vi "RT Main and Scoreboard.vi"() -> ()   [LabVIEW 2026]
uses:
  RT Image.ctl
  RT States.ctl
  Idle Pattern.ctl
  Score.ctl
  SideSelector.ctl
  RT Commands.ctl
  Game Settings.ctl
  2 Player Bitfile dynRef.ctl
  <vilib>/FPGAPlugInAG/cRIO-9047/niLvFpga_Open_cRIO-9047.vi
  <vilib>/rvi/interface/common/dynamic/niFpgaDynamicAddResources.vi
  <vilib>/FPGAPlugInAG/Dynamic/niLvFpga_Run_Dynamic.vi
  <vilib>/Utility/error.llb/Error Cluster From Error Code.vi
  <vilib>/rvi/errors/niLvFpgaAdjustHostInterfaceError.vi
  <vilib>/FPGAPlugInAG/Dynamic/niLvFpga_Abort_Dynamic.vi
  <vilib>/FPGAPlugInAG/Dynamic/niLvFpga_Close_Dynamic.vi
  <vilib>/rvi/interface/nirviOpenFPGA/nirviOpenFPGA.xnode
  FPGA Bitfiles/speedofvight_IdlePattern.lvbitx
  <vilib>/rvi/interface/nirviMethod/nirviMethod.xnode
  <vilib>/rvi/interface/nirviReadWriteControl/nirviReadWriteControl.xnode
  <vilib>/rvi/interface/nirviCloseFPGA/nirviCloseFPGA.xnode
  FPGA Bitfiles/speedofvight_1Player.lvbitx
  FPGA Bitfiles/speedofvight_2Player.lvbitx
  <vilib>/rvi/interface/Simulation/niFpgaSimulationCallBeginRW.vi
  NiFpgaLv.dll
  <vilib>/Utility/Data Type/NI_Data Type.lvlib
panel:
  out "error out 3":errorcluster
  out "error out 2":errorcluster
  out "x-y*floor(x/y)":u32
  out "floor(x/y)":u32
  in  "Winner Display time, ms":u32=7000
  in  "2 Players":bool
  in  "Idle Pattern Cycle Time":u32=5000
  in  "abort":bool
  in  "End Idle":bool
  out "error out":errorcluster
  in  "Speed Threshold, ticks":u64=3000
  in  "Debounce Threshold, ticks":u64=5000
  in  "Game Time":u32=4
  in  "End Game":bool
  out "Score P1":u16 format="%03.0f"
  out "Score P2":u16 format="%03.0f"
  out "2D Picture":T1
  out "Time Remaining":u32 format="%03.0f"
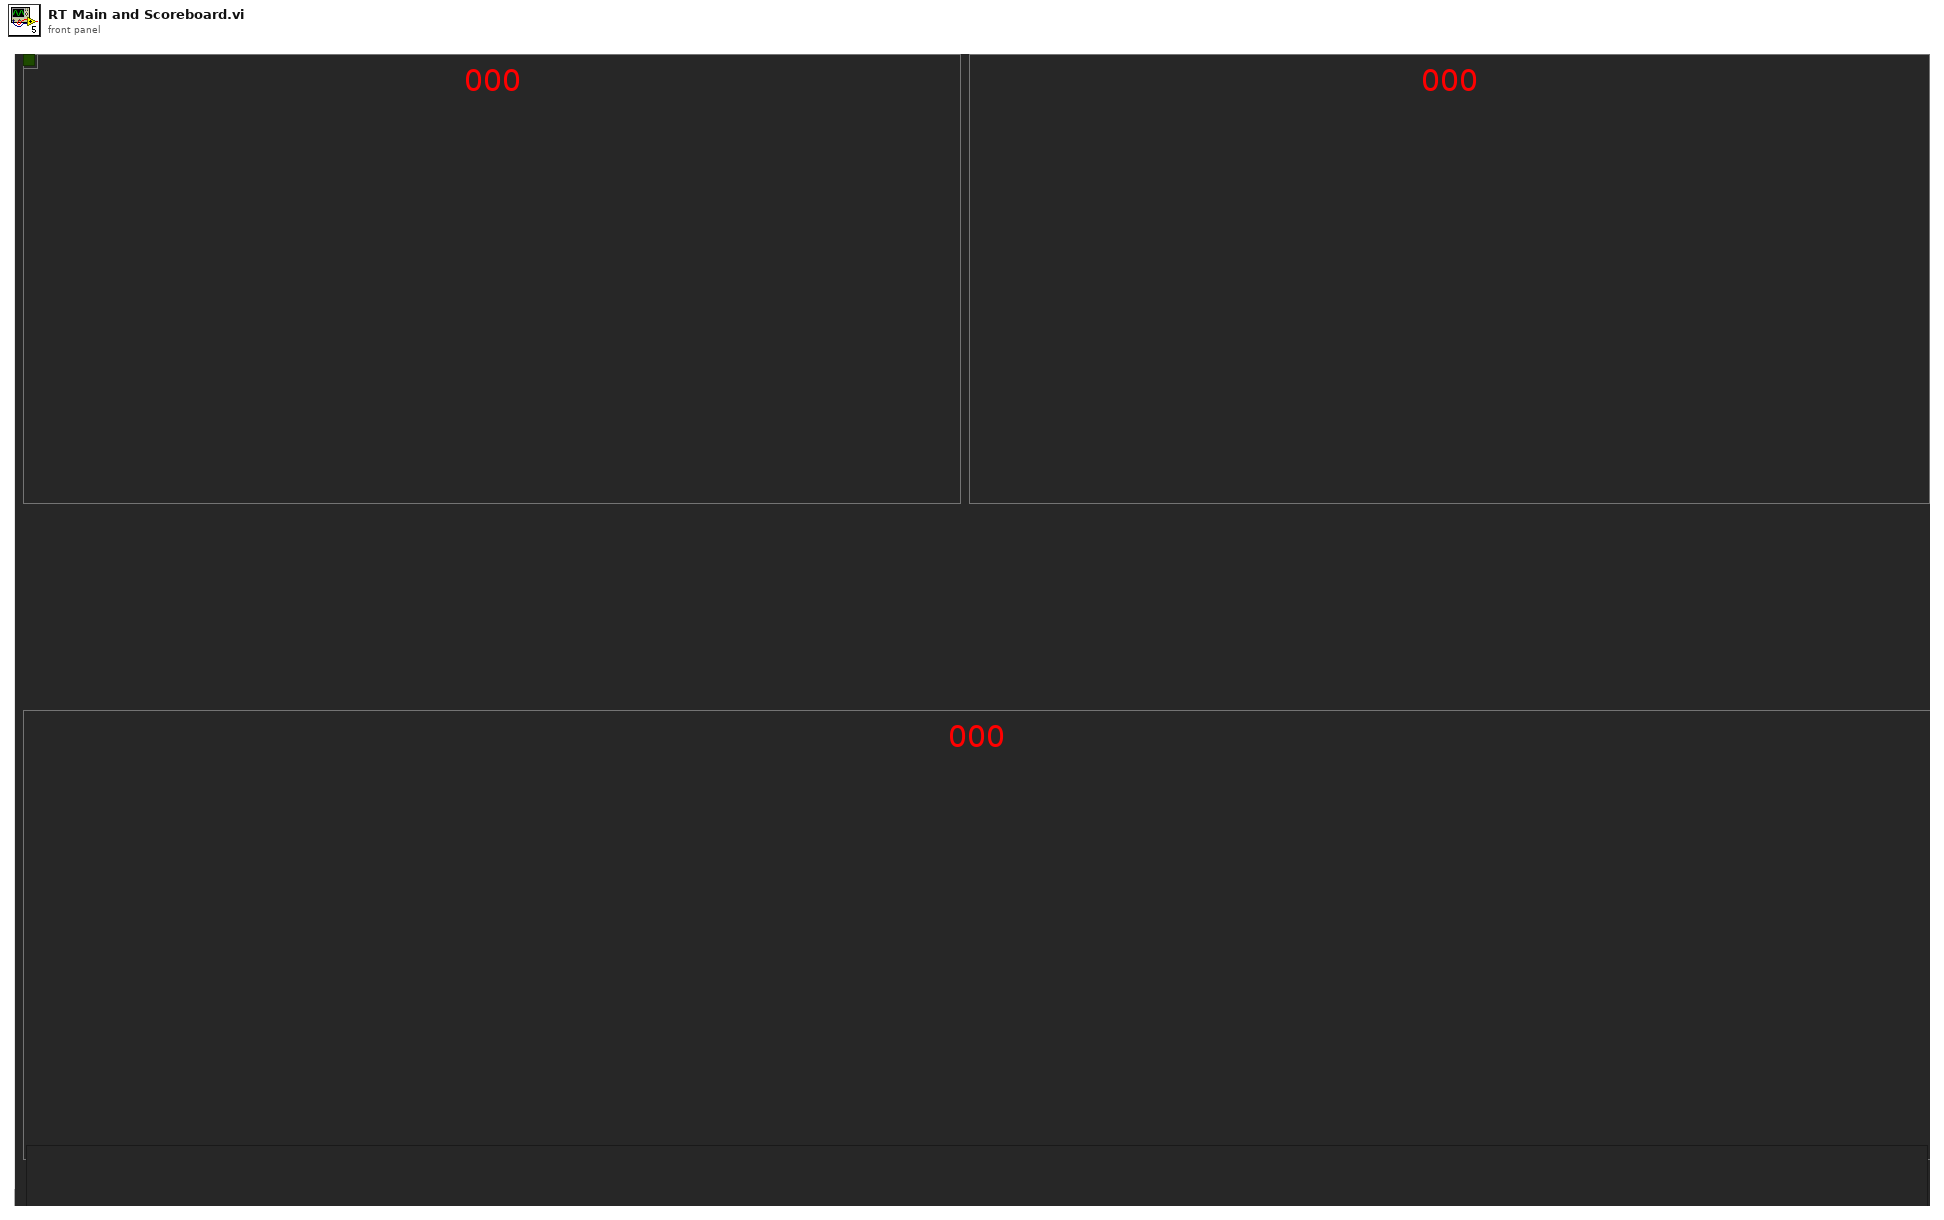
[diagram p1: front panel]
types:
  T1 = typedef "RT Image.ctl" = picture
  T2 = typedef "Score.ctl" = cluster{"Score P1":u16, "Score P2":u16, "Winner Selection":T3}
  T3 = typedef "SideSelector.ctl" = enum16{"P12", "P1", "P2"}
  T4 = cluster{"Debounce Threshold, ticks":u64, "Speed Threshold, ticks":u64, "Game Time":u32, "Idle Pattern Cycle Time, ms":u32, "Winner Display time, ms":u32, "Final Score":T2}
  T5 = typedef "Idle Pattern.ctl" = enum16{"Expanding Circle", "Plasma", "Radar Sweep", "Matrix Rain", "Campfire", "Diagonal Scan"}
  T6 = typedef "RT States.ctl" = enum16{"Idle", "Configuring", "1Player", "2Player", "Display Winner"}
  T7 = typedef "RT Commands.ctl" = enum16{"<null>", "End Idle", "Reset", "Commit Settings", "Commit Host Settings"}
  T8 = typedef "2 Player Bitfile dynRef.ctl" = refnum<k20>
  T9 = typedef "Game Settings.ctl" = cluster{"Speed Threshold, ticks":u64, "Game Time":u32, "2 Players":bool}
  T10 = cluster{"Score P1":u16, "Score P2":u16, "Winner Selection":T3}
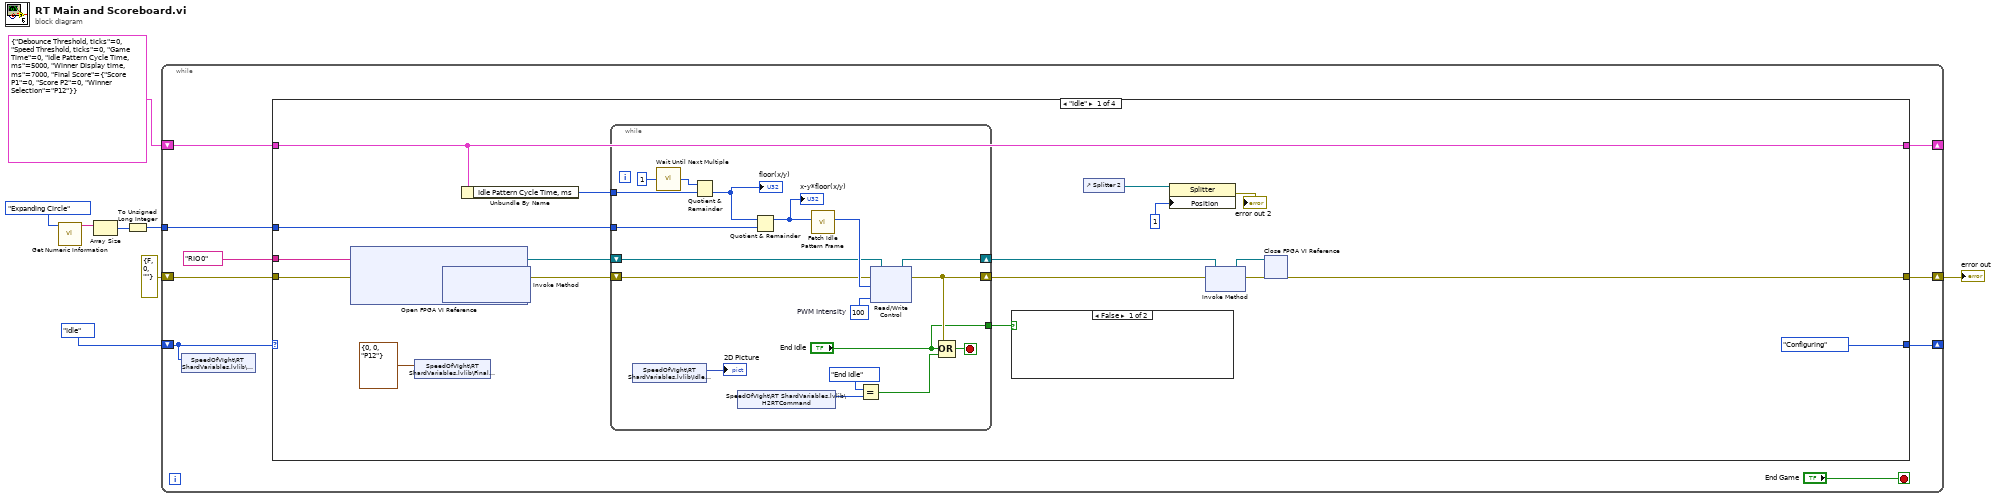
[diagram p0: block diagram]
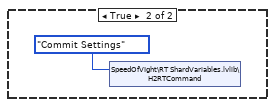
[diagram p2: hidden frame]
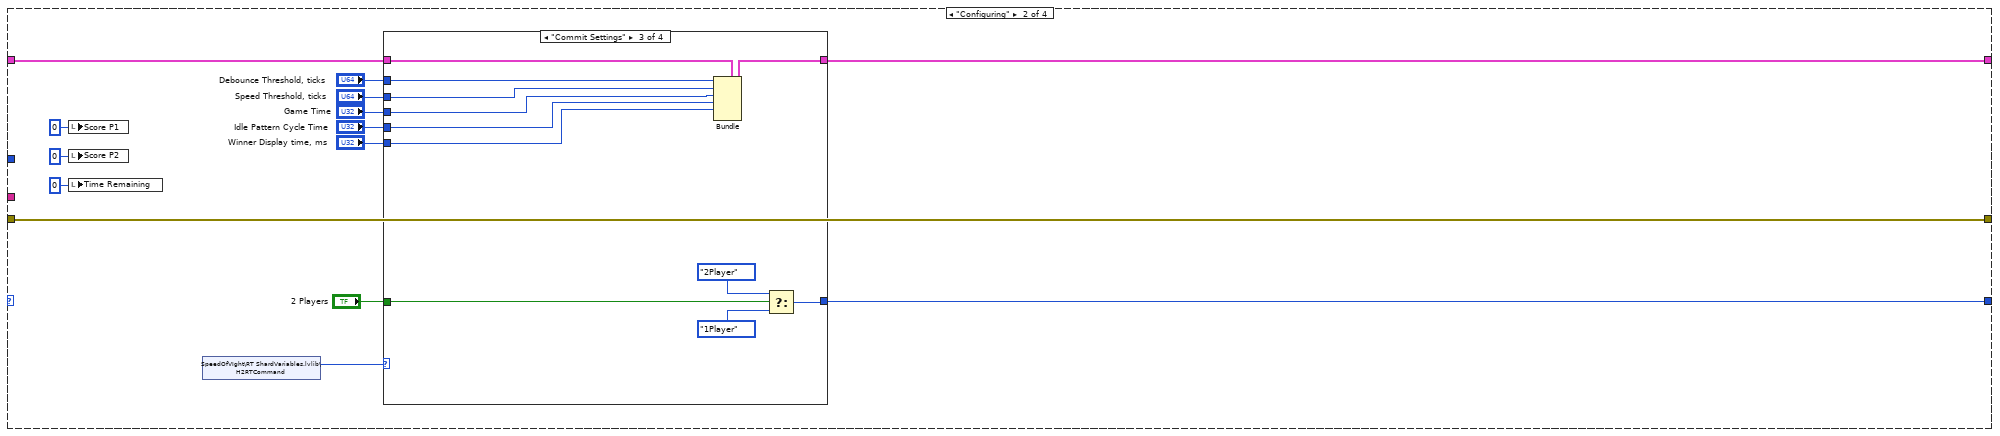
[diagram p3: hidden frame]
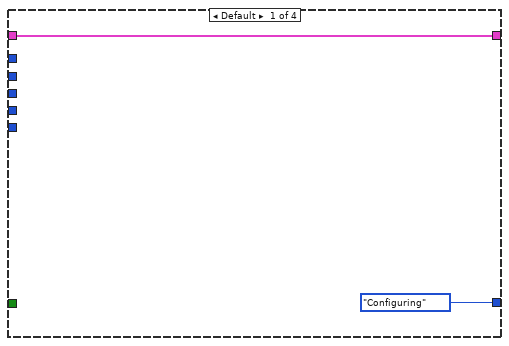
[diagram p4: hidden frame]
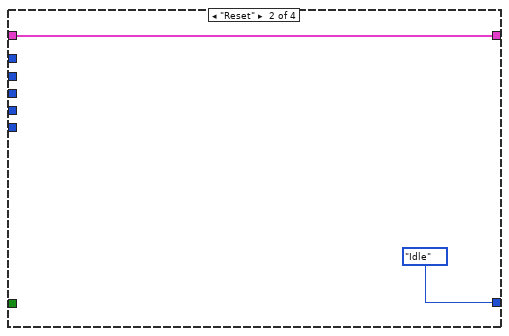
[diagram p5: hidden frame]
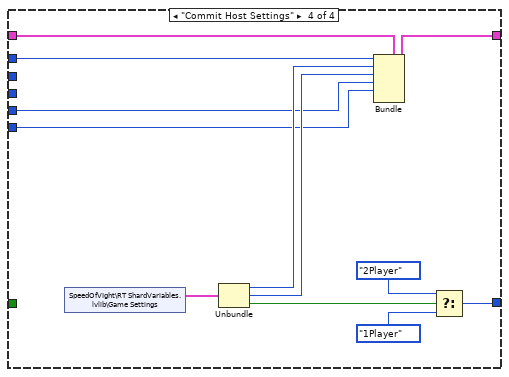
[diagram p6: hidden frame]
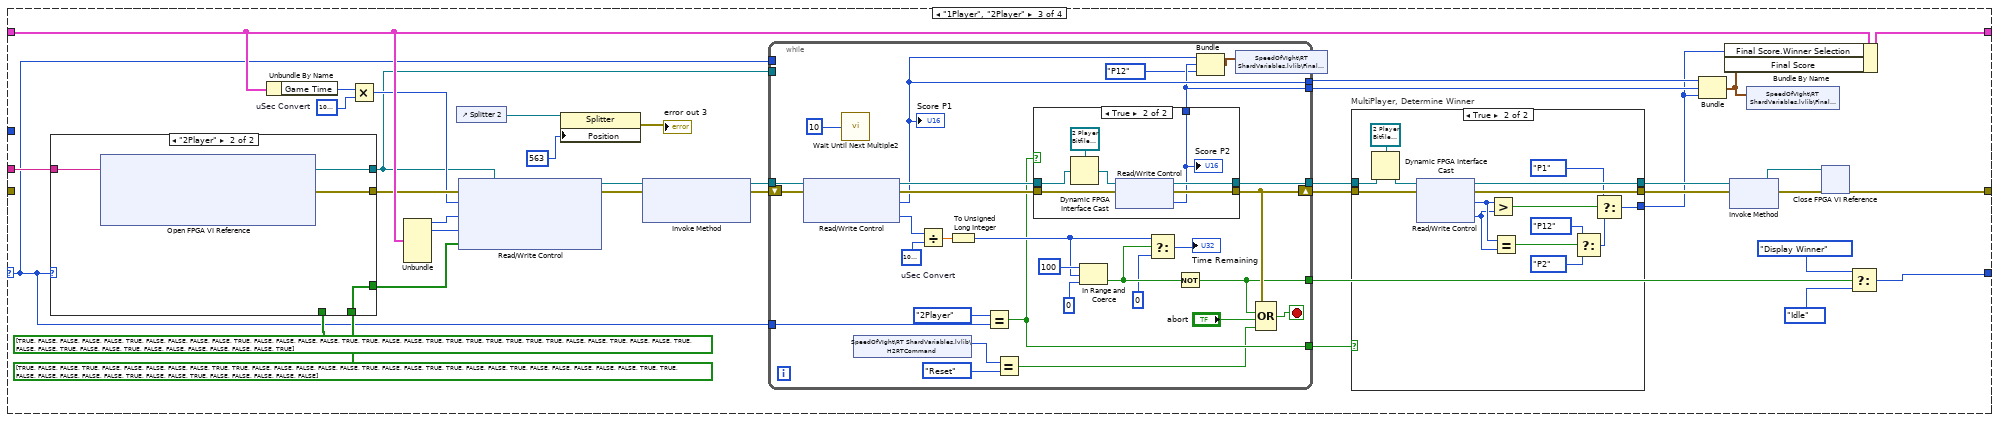
[diagram p7: hidden frame]
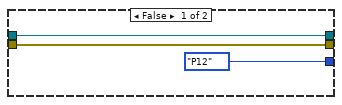
[diagram p8: hidden frame]
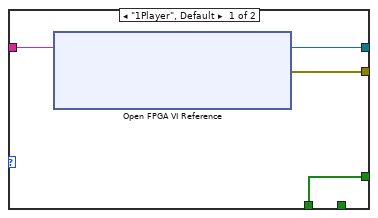
[diagram p9: hidden frame]
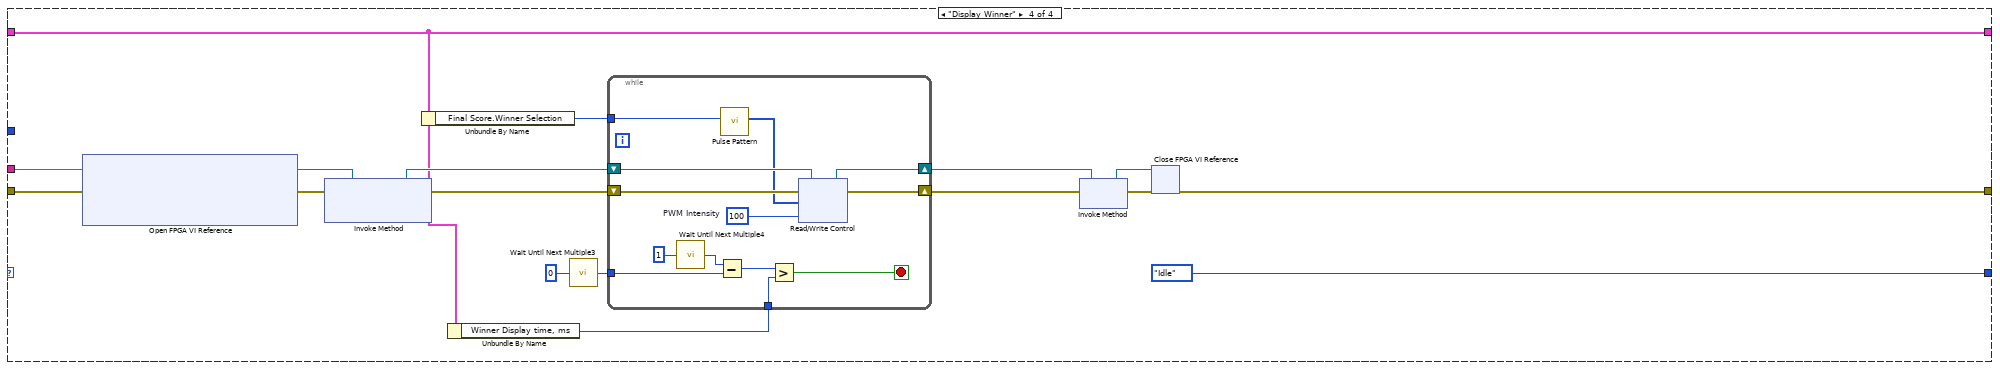
[diagram p11: hidden frame]
diagram:
  n1 = call <vilib>:"Get Numeric Information.vi"("variant"=Idle_Pattern."Expanding Circle" ("Effect")) -> ("enum names"=w6:string[])  [unwired: 7 in, 3 out]
  n2 = Array Size(array=w6) -> (size(s)=w5:i32)
  n3 = To Unsigned Long Integer(number=w5) -> (unsigned 32bit integer=w1:u32)
  n4 = while {
    shift-right: [w13] -> _
    shift-left: RT_States."Idle" ("Enum") -> [w10]
    tunnel: w1 -> [w16]
    shift-right: [w15] -> w4
    shift-left: errorcluster {"status"=FALSE, "code"=0, "source"=""} ("error out") -> [w14]
    shift-right: [w11] -> _
    shift-left: T4 {"Debounce Threshold, ticks"=0, "Speed Threshold, ticks"=0, "Game Time"=0, "Idle Pattern Cycle Time, ms"=5000, "Winner Display time, ms"=7000, "Final Score"={"Score P1"=0, "Score P2"=0, "Winner Selection"=enum."P12"}} ("cluster") -> [w12]
    stop <- "End Game" stop-if-true
    n5 = shared-variable "SpeedOfVIght\\RT ShardVariables.lvlib\\RT2HState"(w10) -> ()  [unwired: 1 in, 1 out]
    n6 = case shown="\"Idle\"" w10 {
      selector: w10 -> [_ _ w103 _]
      tunnel: tag "RIO0" ("resource name") -> [w33 _ w126 w211]
      tunnel: w16 -> [w32 _ _ _]
      tunnel: [w27 w70 w120 w206] -> w15
      tunnel: w14 -> [w26 w70 _ w205]
      tunnel: [RT_States."Configuring" ("Enum") w67 w113 RT_States."Idle" ("Enum")] -> w13
      tunnel: w12 -> [w23 w69 w134 w199]
      tunnel: [w23 w68 w114 w199] -> w11
      frame "Idle" {
        n7 = xnode "Open FPGA VI Reference"("error in"=w26, "resource name"=w33) -> ("FPGA VI Reference Out"=w35:refnum<k20>, "error out"=w37:errorcluster)
        n8 = shared-variable "SpeedOfVIght\\RT ShardVariables.lvlib\\Final Score"(T2 {"Score P1"=0, "Score P2"=0, "Winner Selection"=enum."P12"} ("Final Score")) -> ()  [unwired: 1 in, 1 out]
        n9 = xnode "Invoke Method"("FPGA VI Reference In"=w35, "error in"=w37) -> ("FPGA VI Reference Out"=w34:refnum<k20>, "error out"=w36:errorcluster)  [unwired: 1 in]
        n10 = Unbundle By Name(w23) -> ("Idle Pattern Cycle Time, ms"=w24:u32)
        n11 = while {
          shift-right: [w47] -> w29
          shift-left: w36 -> [w54]
          shift-right: [w52] -> w28
          shift-left: w34 -> [w53]
          tunnel: w32 -> [w45]
          tunnel: w24 -> [w46]
          tunnel: ["End Idle"] -> w22
          stop <- w50 stop-if-true
          w55 = u16 100  # PWM Intensity
          n12 = shared-variable "SpeedOfVIght\\RT ShardVariables.lvlib\\Idle Image"() -> (→"2D Picture":T1)  [unwired: 1 in, 1 out]
          n13 = call "Wait Until Next Multiple"("Count(mSec)"=u32 1 ("Count(Ticks)")) -> ("Tick Count(mSec)"=w42:u32)
          n14 = Quotient & Remainder(x=w42, y=w46) -> (floor(x/y)=w44:u32)  [unwired: 1 out]
          "floor(x/y)" <- w44
          n15 = shared-variable "SpeedOfVIght\\RT ShardVariables.lvlib\\H2RTCommand"() -> (w41:T7)  [unwired: 1 in, 1 out]
          n16 = Quotient & Remainder(x=w44, y=w45) -> (x-y*floor(x/y)=w43:u32)  [unwired: 1 out]
          "x-y*floor(x/y)" <- w43
          n17 = call "Fetch Idle Pattern Frame.vi"("Effect"=w43) -> ("Array"=w56:u16[])  [unwired: 10 in]
          n18 = Equal?(x=RT_Commands."End Idle", y=w41) -> (x = y?=w48:bool)
          n19 = xnode "Read/Write Control"("FPGA VI Reference In"=w53, "error in"=w54, "x"=w56, "Period"=w55) -> ("FPGA VI Reference Out"=w52:refnum<k20>, "error out"=w47:errorcluster)
          n20 = Compound Arithmetic op=OR(w47, "End Idle", w48) -> (w50:bool)
        }
        n21 = case shown="False" w22 {
          frame False {
          }
          frame True {
            n22 = shared-variable "SpeedOfVIght\\RT ShardVariables.lvlib\\H2RTCommand"(RT_Commands."Commit Settings" ("H2RTCommand")) -> ()  [unwired: 1 in, 1 out]
          }
        }
        n23 = control-ref of="Splitter 2"() -> (w20:refnum<vi>)
        n24 = property class="Splitter"(reference=w20, "Position"=1 ("Splitter Position")) -> (error out=→"error out 2":errorcluster)  [unwired: 1 in, 1 out]
        n25 = xnode "Invoke Method"("FPGA VI Reference In"=w28, "error in"=w29) -> ("FPGA VI Reference Out"=w31:refnum<k20>, "error out"=w30:errorcluster)
        n26 = xnode "Close FPGA VI Reference"("FPGA VI Reference In"=w31, "error in"=w30) -> ("error out"=w27:errorcluster)
      }
      frame "Configuring" {
        n27 = local write "Score P1"(u16 0 ("Score P1")) -> ()
        n28 = local write "Score P2"(u16 0 ("Score P2")) -> ()
        n29 = local write "Time Remaining"(u32 0 ("Time Remaining")) -> ()
        n30 = shared-variable "SpeedOfVIght\\RT ShardVariables.lvlib\\H2RTCommand"() -> (w63:T7)  [unwired: 1 in, 1 out]
        n31 = case shown="\"Commit Settings\"" w63 {
          tunnel: w69 -> [w71 w74 w83 w95]
          tunnel: [w71 w74 w82 w94] -> w68
          tunnel: [RT_States."Configuring" ("Enum") RT_States."Idle" ("Enum") w81 w93] -> w67
          tunnel: "Winner Display time, ms" -> [_ _ w75 w86]
          tunnel: "Idle Pattern Cycle Time" -> [_ _ w76 w87]
          tunnel: "Speed Threshold, ticks" -> [_ _ w80 _]
          tunnel: "Debounce Threshold, ticks" -> [_ _ w79 w92]
          tunnel: "Game Time" -> [_ _ w78 _]
          tunnel: "2 Players" -> [_ _ w77 _]
          frame Default {
          }
          frame "Reset" {
          }
          frame "Commit Settings" {
            n32 = Bundle(cluster=w83, "Debounce Threshold, ticks"=w79, "Speed Threshold, ticks"=w80, "Game Time"=w78, "Idle Pattern Cycle Time, ms"=w76, "Winner Display time, ms"=w75) -> (w82:T4)  [unwired: 1 in]
            n33 = Select(t=RT_States."2Player" ("Enum"), s=w77, f=RT_States."1Player" ("Enum")) -> (s? t:f=w81:T6)
          }
          frame "Commit Host Settings" {
            n34 = shared-variable "SpeedOfVIght\\RT ShardVariables.lvlib\\Game Settings"() -> (w91:T9)  [unwired: 1 in, 1 out]
            n35 = Unbundle(w91) -> ("Speed Threshold, ticks"=w90:u64, "Game Time"=w88:u32, "2 Players"=w89:bool)
            n36 = Bundle(cluster=w95, "Debounce Threshold, ticks"=w92, "Speed Threshold, ticks"=w90, "Game Time"=w88, "Idle Pattern Cycle Time, ms"=w87, "Winner Display time, ms"=w86) -> (w94:T4)  [unwired: 1 in]
            n37 = Select(t=RT_States."2Player" ("Enum"), s=w89, f=RT_States."1Player" ("Enum")) -> (s? t:f=w93:T6)
          }
        }
      }
      frame "1Player", "2Player" {
        w133 = u32 1000000  # uSec Convert
        n38 = case shown="\"2Player\"" w103 {
          tunnel: [w156 w160] -> w130
          tunnel: [w155 w159] -> w102
          tunnel: w126 -> [w154 w158]
          tunnel: [w153 w157] -> w101
          tunnel: bool[] [TRUE, FALSE, FALSE, TRUE, FALSE, FALSE, FALSE, FALSE, FALSE, TRUE, TRUE, FALSE, FALSE, FALSE, FALSE, FALSE, TRUE, FALSE, FALSE, TRUE, TRUE, FALSE, FALSE, TRUE, FALSE, FALSE, FALSE, FALSE, FALSE, TRUE, TRUE, FALSE, FALSE, FALSE, FALSE, FALSE, TRUE, FALSE, FALSE, TRUE, FALSE, FALSE, FALSE, FALSE, FALSE] ("appended array") -> [_ w157]
          tunnel: bool[] [TRUE, FALSE, FALSE, FALSE, FALSE, TRUE, FALSE, FALSE, FALSE, FALSE, TRUE, FALSE, FALSE, FALSE, FALSE, TRUE, TRUE, FALSE, FALSE, TRUE, TRUE, TRUE, TRUE, TRUE, TRUE, TRUE, FALSE, FALSE, TRUE, FALSE, FALSE, TRUE, FALSE, FALSE, TRUE, FALSE, FALSE, TRUE, FALSE, FALSE, FALSE, FALSE, FALSE, FALSE, TRUE] ("appended array") -> [w153 _]
          frame "1Player", Default {
            n39 = xnode "Open FPGA VI Reference"("resource name"=w154) -> ("FPGA VI Reference Out"=w155:refnum<k20>, "error out"=w156:errorcluster)  [unwired: 1 in]
          }
          frame "2Player" {
            n40 = xnode "Open FPGA VI Reference"("resource name"=w158) -> ("FPGA VI Reference Out"=w159:refnum<k20>, "error out"=w160:errorcluster)  [unwired: 1 in]
          }
        }
        n41 = Unbundle By Name(w134) -> ("Game Time"=w123:u32)
        n42 = Multiply(x=w123, y=w133) -> (x*y=w127:u32)
        n43 = Unbundle(w134) -> ("Debounce Threshold, ticks"=w125:u64, "Speed Threshold, ticks"=w124:u64)  [unwired: 4 out]
        n44 = control-ref of="Splitter 2"() -> (w100:refnum<vi>)
        n45 = xnode "Read/Write Control"("FPGA VI Reference In"=w102, "error in"=w130, "Game Time, uS"=w127, "Debounce Threshold, ticks"=w125, "Speed Threshold, ticks"=w124, "Starting Lights"=w101) -> ("FPGA VI Reference Out"=w128:refnum<k20>, "error out"=w129:errorcluster)
        n46 = property class="Splitter"(reference=w100, "Position"=563 ("Splitter Position")) -> (error out=→"error out 3":errorcluster)  [unwired: 1 in, 1 out]
        n47 = xnode "Invoke Method"("FPGA VI Reference In"=w128, "error in"=w129) -> ("FPGA VI Reference Out"=w132:refnum<k20>, "error out"=w131:errorcluster)  [unwired: 1 in]
        n48 = while {
          tunnel: w132 -> [w189]
          shift-right: [w182] -> w117
          shift-left: w131 -> [w188]
          tunnel: w103 -> [w180]
          tunnel: [w176] -> w118
          tunnel: [w169] -> w111
          tunnel: [w168] -> w119
          tunnel: [w164] -> w107
          tunnel: [w163] -> w106
          tunnel: w103 -> [_]
          tunnel: w102 -> [_]
          stop <- w183 stop-if-true
          w186 = u32 1000000  # uSec Convert
          n49 = xnode "Read/Write Control"("FPGA VI Reference In"=w189, "error in"=w188) -> ("FPGA VI Reference Out"=w181:refnum<k20>, "error out"=w184:errorcluster, "Score P1"=w164:u16, "Time Remaining"=w173:u32)
          "Score P1" <- w164
          n50 = call "Wait Until Next Multiple2"("Count(mSec)"=u32 10 ("Count(Ticks)")) -> ()  [unwired: 1 out]
          n51 = shared-variable "SpeedOfVIght\\RT ShardVariables.lvlib\\H2RTCommand"() -> (w165:T7)  [unwired: 1 in, 1 out]
          n52 = Divide(x=w173, y=w186) -> (x/y=w187:dbl)
          n53 = To Unsigned Long Integer(number=w187) -> (unsigned 32bit integer=w170:u32)
          n54 = Equal?(x=RT_States."2Player", y=w180) -> (x = y?=w168:bool)
          n55 = Equal?(x=w165, y=RT_Commands."Reset") -> (x = y?=w166:bool)
          n56 = case shown="True" w168 {
            tunnel: w184 -> [w191 w198]
            tunnel: [w191 w197] -> w182
            tunnel: w181 -> [w190 w195]
            tunnel: [w190 w193] -> w176
            tunnel: [_ w192] -> w163
            frame False {
            }
            frame True {
              n57 = Dynamic FPGA Interface Cast(Session In=T8 refnum ("FPGA Interface"), Type=w195) -> (Session Out=w194:T8)
              n58 = xnode "Read/Write Control"("FPGA VI Reference In"=w194, "error in"=w198) -> ("FPGA VI Reference Out"=w193:T8, "error out"=w197:errorcluster, "Score P2"=w192:u16)
              "Score P2" <- w192
            }
          }
          n59 = In Range and Coerce(upper limit=u32 100, x=w170, lower limit=u32 0 ("y")) -> (In Range?=w174:bool)  [unwired: 1 out]
          n60 = Select(t=w170, s=w174, f=u32 0 ("y")) -> (s? t:f=→"Time Remaining":u32)
          n61 = Not(x=w174) -> (.not. x?=w169:bool)
          n62 = Bundle("Score P1"=w164, "Score P2"=w163, "Winner Selection"=SideSelector."P12") -> (w161:T10)  [unwired: 1 in]
          n63 = shared-variable "SpeedOfVIght\\RT ShardVariables.lvlib\\Final Score"(w161) -> ()  [unwired: 1 in, 1 out]
          n64 = Compound Arithmetic op=OR(w182, w169, "abort", w166) -> (w183:bool)
        }
        n65 = case "MultiPlayer, Determine Winner" shown="True" w119 {
          tunnel: w118 -> [w136 w148]
          tunnel: w117 -> [w137 w152]
          tunnel: [w137 w151] -> w116
          tunnel: [w136 w150] -> w115
          tunnel: [SideSelector."P12" ("Winner Selection") w143] -> w104
          frame False {
          }
          frame True {
            n66 = Dynamic FPGA Interface Cast(Session In=T8 refnum ("FPGA Interface"), Type=w148) -> (Session Out=w149:T8)
            n67 = xnode "Read/Write Control"("FPGA VI Reference In"=w149, "error in"=w152) -> ("FPGA VI Reference Out"=w150:T8, "error out"=w151:errorcluster, "Score P1"=w146:u16, "Score P2"=w142:u16)
            n68 = Greater?(x=w146, y=w142) -> (0:w147:bool)
            n69 = Equal?(x=w146, y=w142) -> (x = y?=w145:bool)
            n70 = Select(t=SideSelector."P12" ("Winner Selection"), s=w145, f=SideSelector."P2" ("Winner Selection")) -> (s? t:f=w139:T3)
            n71 = Select(t=SideSelector."P1" ("Winner Selection"), s=w147, f=w139) -> (s? t:f=w143:T3)
          }
        }
        n72 = Bundle("Score P1"=w107, "Score P2"=w106, "Winner Selection"=w104) -> (w105:T10)  [unwired: 1 in]
        n73 = Bundle By Name(cluster=w134, "Final Score.Winner Selection"=w104, "Final Score"=w105) -> (w114:T4)
        n74 = xnode "Invoke Method"("FPGA VI Reference In"=w115, "error in"=w116) -> ("FPGA VI Reference Out"=w122:refnum<k20>, "error out"=w121:errorcluster)
        n75 = shared-variable "SpeedOfVIght\\RT ShardVariables.lvlib\\Final Score"(w105) -> ()  [unwired: 1 in, 1 out]
        n76 = xnode "Close FPGA VI Reference"("FPGA VI Reference In"=w122, "error in"=w121) -> ("error out"=w120:errorcluster)
        n77 = Select(t=RT_States."Display Winner" ("Enum"), s=w111, f=RT_States."Idle" ("Enum")) -> (s? t:f=w113:T6)
      }
      frame "Display Winner" {
        n78 = xnode "Open FPGA VI Reference"("error in"=w205, "resource name"=w211) -> ("FPGA VI Reference Out"=w213:refnum<k20>, "error out"=w215:errorcluster)
        n79 = xnode "Invoke Method"("FPGA VI Reference In"=w213, "error in"=w215) -> ("FPGA VI Reference Out"=w212:refnum<k20>, "error out"=w214:errorcluster)  [unwired: 1 in]
        n80 = Unbundle By Name(w199) -> ("Final Score.Winner Selection"=w203:T3)
        n81 = Unbundle By Name(w199) -> ("Winner Display time, ms"=w200:u32)
        n82 = call "Wait Until Next Multiple3"("Count(mSec)"=u32 0 ("Count(Ticks)")) -> ("Tick Count(mSec)"=w201:u32)
        n83 = while {
          shift-right: [w228] -> w208
          shift-left: w214 -> [w226]
          shift-right: [w224] -> w207
          shift-left: w212 -> [w225]
          tunnel: w203 -> [w223]
          tunnel: w201 -> [w219]
          tunnel: w200 -> [w217]
          stop <- w216 stop-if-true
          w227 = u16 100  # PWM Intensity
          n84 = call "Wait Until Next Multiple4"("Count(mSec)"=u32 1 ("Count(Ticks)")) -> ("Tick Count(mSec)"=w220:u32)
          n85 = Subtract(x=w220, y=w219) -> (x-y=w218:u32)
          n86 = call "Pulse Pattern.vi"("Selector"=w223) -> ("Array"=w222:u16[])  [unwired: 10 in]
          n87 = Greater?(x=w218, y=w217) -> (0:w216:bool)
          n88 = xnode "Read/Write Control"("FPGA VI Reference In"=w225, "error in"=w226, "x"=w222, "Period"=w227) -> ("FPGA VI Reference Out"=w224:refnum<k20>, "error out"=w228:errorcluster)
        }
        n89 = xnode "Invoke Method"("FPGA VI Reference In"=w207, "error in"=w208) -> ("FPGA VI Reference Out"=w210:refnum<k20>, "error out"=w209:errorcluster)
        n90 = xnode "Close FPGA VI Reference"("FPGA VI Reference In"=w210, "error in"=w209) -> ("error out"=w206:errorcluster)
      }
    }
  }
  "error out" <- w4
